vi "SOFandEOF.vi"(8 "error in (no error)":errorcluster, 11 "ISO 14443 A UP in":refnum<class "ISO 14443 A UP.lvclass">) -> (0 "error out":errorcluster, 3 "ISO 14443 A UP out":refnum<class "ISO 14443 A UP.lvclass">, 5 "frame":u8[](array[numeric]))   [LabVIEW 2019, in "ISO 14443 A UP.lvclass"]
uses:
  ISO 14443 A UP.lvclass
  TypeDef/Store.ctl
  ISO 14443 A UP.lvclass/ISO 14443 A UP.ctl
  RFID system.lvclass
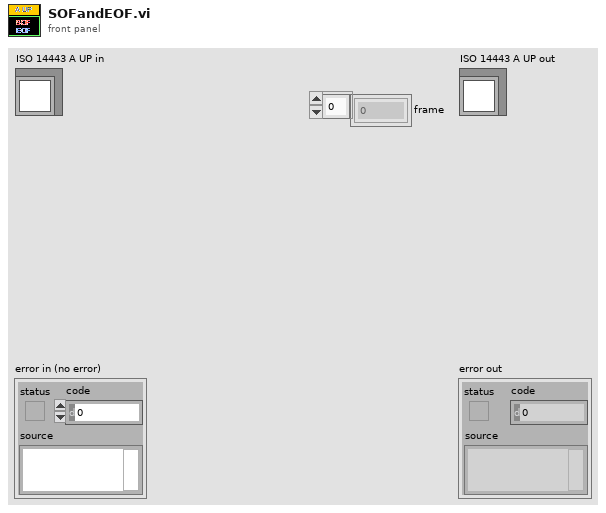
[diagram p1: front panel]
types:
  T1 = typedef "Store.ctl" = enum16{"envelope", "noise", "demSubCar", "CH_frame", "Decode", "demodulate", "in", "out", "sum", "subCarrier", "frame", "command", "encode", "modulate", "encode_UP", "modulate_up", "demod_up", "envelop_up", "sum_up", "out_up", "in_up"}
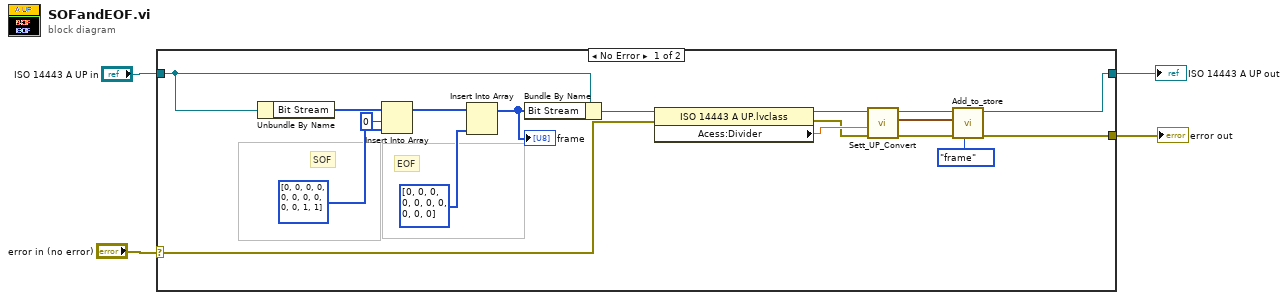
[diagram p0: block diagram]
diagram:
  n1 = case shown="No Error" "error in (no error)" {
    selector: "error in (no error)" -> [w7 w23]
    tunnel: [w16 w24] -> w2
    tunnel: "ISO 14443 A UP in" -> [w17 w24]
    tunnel: [w15 w23] -> w1
    frame No Error {
      # "EOF"
      # "SOF"
      n2 = Unbundle By Name(w17) -> ("Bit Stream"=w18:u8[])
      n3 = Insert Into Array(array=w18, index=0, new element=u8[] [0, 0, 0, 0, 0, 0, 0, 0, 0, 0, 1, 1] ("Bit stream out (NRZ encode)")) -> (w20:u8[])
      n4 = Insert Into Array(array=w20, new element=u8[] [0, 0, 0, 0, 0, 0, 0, 0, 0, 0] ("Bit stream out (NRZ encode)")) -> (w5:u8[])  [unwired: 1 in]
      "frame" <- w5
      n5 = Bundle By Name(cluster=w17, "Bit Stream"=w5) -> (w14:refnum<class "ISO 14443 A UP.lvclass">)
      n6 = property class="ISO 14443 A UP.lvclass"(reference=w14, error in=w7) -> (reference out=w9:refnum<class "ISO 14443 A UP.lvclass">, error out=w6:errorcluster, "Acess:Divider"=w8:dbl)
      n7 = call-dynamic "Sett_UP_Convert.vi"("error in (no error)"=w6, "Divider(1)"=w8, "ISO 14443 A UP in"=w9) -> ("error out"=w11:errorcluster, "Waveform"=w12:waveform(dbl), "ISO 14443 A UP out"=w13:refnum<class "ISO 14443 A UP.lvclass">)  [unwired: 6 in]
      n8 = call "Add_to_store.vi"("Store"=Store."frame", "error in (no error)"=w11, "Waveform"=w12, "RFID system in"=w13) -> ("error out"=w15:errorcluster, "RFID system out"=w16:refnum<class "ISO 14443 A UP.lvclass">)  [unwired: 6 in]
    }
    frame Error {
    }
  }
  "error out" <- w1
  "ISO 14443 A UP out" <- w2
